vi "set presync pulses.vi"(8 "error in (no error)":errorcluster, 11 "DAQOrcaFlash in":refnum<class "DAQOrcaFlash.lvclass">) -> (0 "error out":errorcluster, 3 "DAQOrcaFlash out":refnum<class "DAQOrcaFlash.lvclass">)   [LabVIEW 2012, in "DAQOrcaFlash.lvclass"]
uses:
  DAQOrcaFlash.lvclass
  DAQOrcaFlash.lvclass/DAQOrcaFlash.ctl
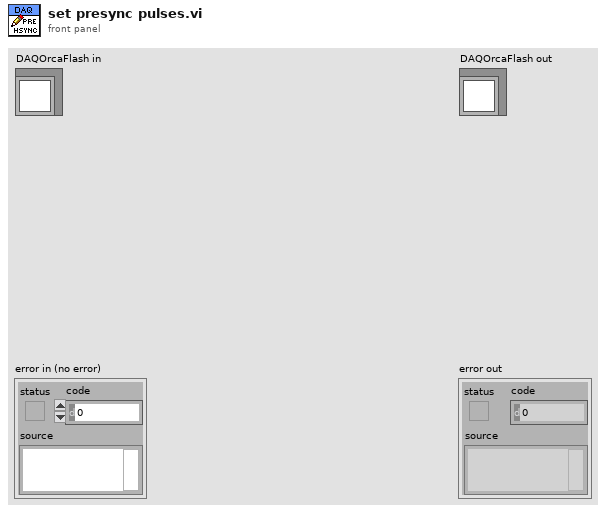
[diagram p1: front panel]
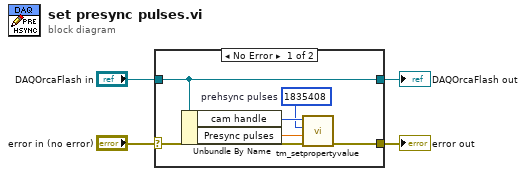
[diagram p0: block diagram]
diagram:
  n1 = case shown="No Error" "error in (no error)" {
    selector: "error in (no error)" -> [w9 w12]
    tunnel: [w8 w12] -> w3
    tunnel: [w10 w11] -> w1
    tunnel: "DAQOrcaFlash in" -> [w10 w11]
    frame No Error {
      w5 = u32 1835408  # prehsync pulses
      n2 = Unbundle By Name(w10) -> ("cam handle"=w7:u32, "Presync pulses"=w6:dbl)
      n3 = call <userlib>:"tm_setpropertyvalue.vi"("error in (no error)"=w9, "Value in"=w6, "Property ID"=w5, "Handle in"=w7) -> ("error out"=w8:errorcluster)  [unwired: 6 in, 1 out]
    }
    frame Error {
    }
  }
  "error out" <- w3
  "DAQOrcaFlash out" <- w1
